vi "Thorlabs Translation Stage Module.vi"(7 "Action":T1, 8 "error in (no error)":errorcluster, 9 "Cluster In":T3, 10 "Set/Get":T2, 11 ".NET Refnum in":refnum<k24>) -> (0 "error out":errorcluster, 2 "Cluster out":T3, 3 ".NET Refnum out":refnum<k24>)   [LabVIEW 2018]
uses:
  C:/Project/SerialSectOCT/SerialSectOCT/Software/Thorlabs.MotionControl.Controls.dll
  Thorlabs.MotionControl.Controls.dll
  Hardware Mfg/Thorlabs Translation Stages/Controls/Translation Stage Cluster.ctl
  Controls/Translation Stage Types.ctl
  Controls/Set Get Controls.ctl
  Hardware Mfg/Thorlabs Translation Stages/Controls/Motion Translation Module Control.ctl
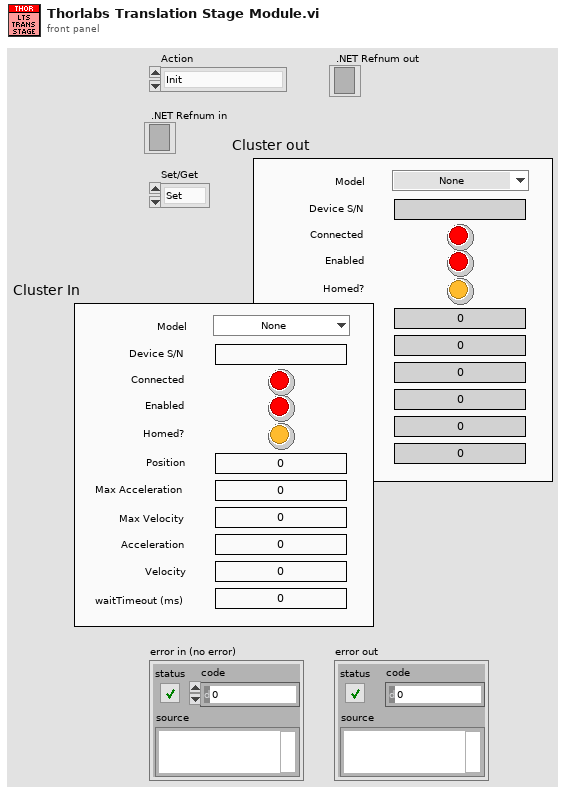
[diagram p1: front panel]
types:
  T1 = typedef "Motion Translation Module Control.ctl" = enum16{"Init", "Home", "Status", "Velocity/Accel", "Position", "Jog", "Stop", "Uninit", "Enable", "Disable"}
  T2 = typedef "Set Get Controls.ctl" = enum16{"Set", "Get"}
  T3 = typedef "Translation Stage Cluster.ctl" = cluster{"Position":dbl, "Is.Enabled?":bool, "Is.Connected?":bool, "Device SN":string, "AccelerationMaximum":dbl, "VelocityMaximum":dbl, "Acceleration":dbl, "Velocity":dbl, "waitTimeout (ms)":i32, "Model":T4, "Is.Homed?":bool}
  T4 = typedef "Translation Stage Types.ctl" = enum16{"None", "Thorlabs LTS", "Thorlabs MLJ"}
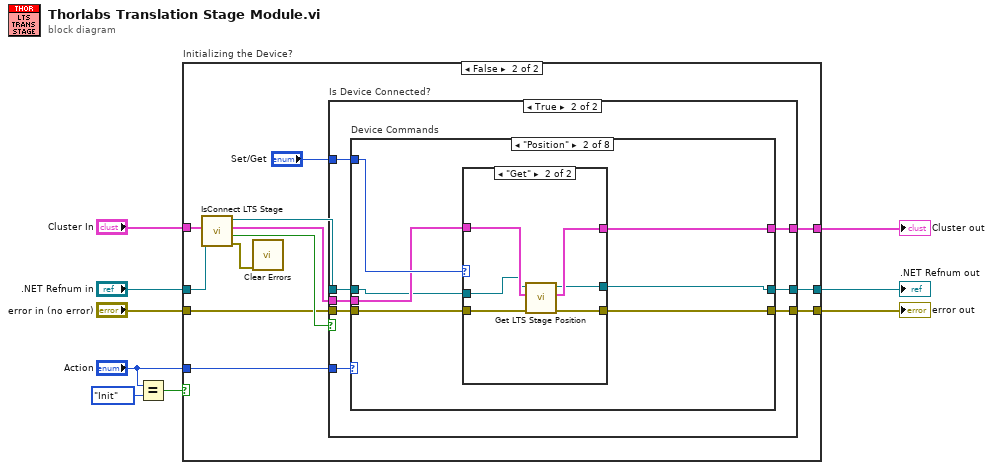
[diagram p0: block diagram]
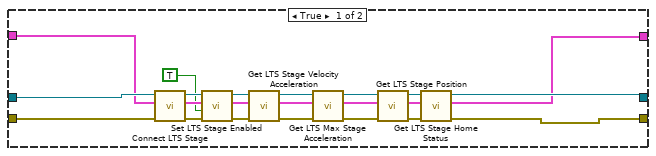
[diagram p2: hidden frame]
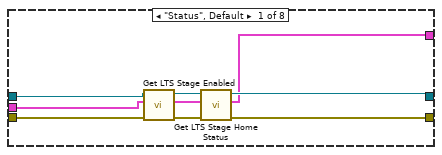
[diagram p4: hidden frame]
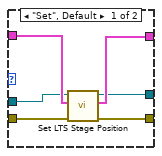
[diagram p5: hidden frame]
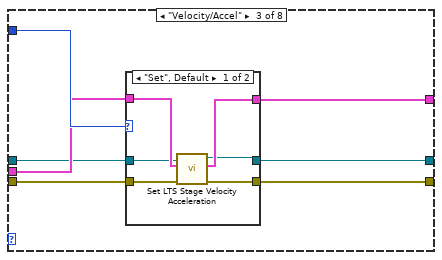
[diagram p6: hidden frame]
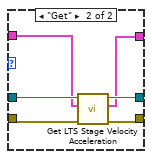
[diagram p7: hidden frame]
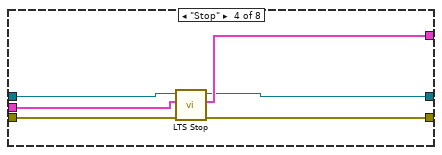
[diagram p8: hidden frame]
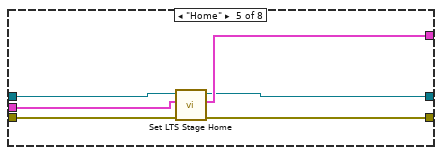
[diagram p9: hidden frame]
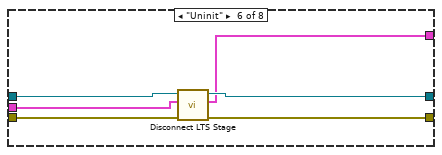
[diagram p10: hidden frame]
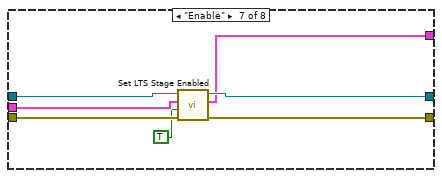
[diagram p11: hidden frame]
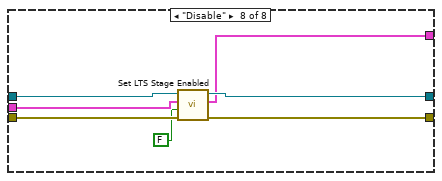
[diagram p12: hidden frame]
diagram:
  n1 = Equal?(x="Action", y=Motion_Translation_Module_Control."Init") -> (x = y?=w1:bool)
  n2 = case "Initializing the Device?" shown="False" w1 {
    tunnel: ".NET Refnum in" -> [w31 w38]
    tunnel: [w19 w43] -> w8
    tunnel: [w18 w42] -> w7
    tunnel: [w11 w41] -> w6
    tunnel: "error in (no error)" -> [w10 w33]
    tunnel: "Cluster In" -> [w30 w35]
    tunnel: "Action" -> [_ w40]
    frame True {
      n3 = call "Connect LTS Stage.vi"("error in (no error)"=w10, "Cluster in"=w30, "LTS Reference In"=w31) -> ("error out"=w29:errorcluster, "Cluster out"=w27:T3, "LTS Reference Out"=w28:refnum<k24>)  [unwired: 5 in, 1 out]
      n4 = call "Set LTS Stage Enabled.vi"("error in (no error)"=w29, "Enable?"=TRUE, "Cluster in"=w27, "LTS Reference In"=w28) -> ("error out"=w26:errorcluster, "Cluster out"=w25:T3, "LTS Reference Out"=w24:refnum<k24>)  [unwired: 5 in]
      n5 = call "Get LTS Stage Velocity Acceleration.vi"("error in (no error)"=w26, "Cluster in"=w25, "LTS Reference In"=w24) -> ("error out"=w23:errorcluster, "Cluster out"=w15:T3, "LTS Reference Out"=w14:refnum<k24>)  [unwired: 5 in, 1 out]
      n6 = call "Get LTS Max Stage Acceleration.vi"("error in (no error)"=w23, "Cluster in"=w15, "LTS Reference In"=w14) -> ("error out"=w16:errorcluster, "Cluster out"=w12:T3, "LTS Reference Out"=w13:refnum<k24>)  [unwired: 4 in, 2 out]
      n7 = call "Get LTS Stage Position.vi"("error in (no error)"=w16, "Cluster in"=w12, "LTS Reference In"=w13) -> ("error out"=w22:errorcluster, "Cluster out"=w21:T3, "LTS Reference Out"=w20:refnum<k24>)  [unwired: 5 in, 1 out]
      n8 = call "Get LTS Stage Home Status.vi"("error in (no error)"=w22, "Cluster in"=w21, "LTS Reference In"=w20) -> ("error out"=w11:errorcluster, "Cluster out"=w18:T3, "LTS Reference Out"=w19:refnum<k24>)  [unwired: 6 in]
    }
    frame False {
      n9 = call "IsConnect LTS Stage.vi"("Cluster in"=w35, "LTS Reference In"=w38) -> ("error out"=w32:errorcluster, "IsConnected"=w36:bool, "Cluster out"=w34:T3, "LTS Reference Out"=w37:refnum<k24>)  [unwired: 6 in]
      n10 = call <vilib>:"Clear Errors.vi"("error in (no error)"=w32) -> ()  [unwired: 5 in, 2 out]
      n11 = case "Is Device Connected?" shown="True" w36 {
        tunnel: w37 -> [w44 w54]
        tunnel: [w44 w53] -> w43
        tunnel: [w46 w52] -> w42
        tunnel: [w45 w51] -> w41
        tunnel: w33 -> [w45 w50]
        tunnel: "Set/Get" -> [_ w49]
        tunnel: w40 -> [_ w48]
        tunnel: w34 -> [w46 w47]
        frame False {
        }
        frame True {
          n12 = case "Device Commands" shown="\"Position\"" w48 {
            tunnel: w49 -> [_ w70 w89 _ _ _ _ _]
            tunnel: w47 -> [w56 w67 w86 w105 w111 w116 w123 w130]
            tunnel: w50 -> [w57 w69 w88 w107 w113 w119 w126 w133]
            tunnel: [w60 w65 w84 w103 w109 w117 w124 w131] -> w53
            tunnel: [w61 w68 w87 w106 w112 w118 w125 w132] -> w51
            tunnel: [w58 w66 w85 w104 w110 w115 w122 w129] -> w52
            tunnel: w54 -> [w55 w64 w83 w102 w108 w114 w121 w128]
            frame "Status", Default {
              n13 = call "Get LTS Stage Enabled.vi"("error in (no error)"=w57, "Cluster in"=w56, "LTS Reference In"=w55) -> ("error out"=w63:errorcluster, "Cluster out"=w59:T3, "LTS Reference Out"=w62:refnum<k24>)  [unwired: 5 in, 1 out]
              n14 = call "Get LTS Stage Home Status.vi"("error in (no error)"=w63, "Cluster in"=w59, "LTS Reference In"=w62) -> ("error out"=w61:errorcluster, "Cluster out"=w58:T3, "LTS Reference Out"=w60:refnum<k24>)  [unwired: 6 in]
            }
            frame "Position" {
              n15 = case shown="\"Get\"" w70 {
                tunnel: w69 -> [w76 w82]
                tunnel: [w75 w81] -> w68
                tunnel: w67 -> [w74 w80]
                tunnel: [w73 w79] -> w66
                tunnel: w64 -> [w72 w78]
                tunnel: [w71 w77] -> w65
                frame "Set", Default {
                  n16 = call "Set LTS Stage Position.vi"("error in (no error)"=w76, "Cluster in"=w74, "LTS Reference In"=w72) -> ("error out"=w75:errorcluster, "Cluster out"=w73:T3, "LTS Reference Out"=w71:refnum<k24>)  [unwired: 6 in]
                }
                frame "Get" {
                  n17 = call "Get LTS Stage Position.vi"("error in (no error)"=w82, "Cluster in"=w80, "LTS Reference In"=w78) -> ("error out"=w81:errorcluster, "Cluster out"=w79:T3, "LTS Reference Out"=w77:refnum<k24>)  [unwired: 5 in, 1 out]
                }
              }
            }
            frame "Velocity/Accel" {
              n18 = case shown="\"Set\", Default" w89 {
                tunnel: w88 -> [w95 w101]
                tunnel: [w94 w100] -> w87
                tunnel: w86 -> [w92 w97]
                tunnel: [w93 w96] -> w85
                tunnel: w83 -> [w91 w98]
                tunnel: [w90 w99] -> w84
                frame "Set", Default {
                  n19 = call "Set LTS Stage Velocity Acceleration.vi"("error in (no error)"=w95, "Cluster in"=w92, "LTS Reference In"=w91) -> ("error out"=w94:errorcluster, "Cluster out"=w93:T3, "LTS Reference Out"=w90:refnum<k24>)  [unwired: 6 in]
                }
                frame "Get" {
                  n20 = call "Get LTS Stage Velocity Acceleration.vi"("error in (no error)"=w101, "Cluster in"=w97, "LTS Reference In"=w98) -> ("error out"=w100:errorcluster, "Cluster out"=w96:T3, "LTS Reference Out"=w99:refnum<k24>)  [unwired: 5 in, 1 out]
                }
              }
            }
            frame "Stop" {
              n21 = call "LTS Stop.vi"("error in (no error)"=w107, "Cluster in"=w105, "LTS Reference In"=w102) -> ("error out"=w106:errorcluster, "Cluster out"=w104:T3, "LTS Reference Out"=w103:refnum<k24>)  [unwired: 6 in]
            }
            frame "Home" {
              n22 = call "Set LTS Stage Home.vi"("error in (no error)"=w113, "Cluster in"=w111, "LTS Reference In"=w108) -> ("error out"=w112:errorcluster, "Cluster out"=w110:T3, "LTS Reference Out"=w109:refnum<k24>)  [unwired: 6 in]
            }
            frame "Uninit" {
              n23 = call "Disconnect LTS Stage.vi"("error in (no error)"=w119, "Cluster in"=w116, "LTS Reference In"=w114) -> ("error out"=w118:errorcluster, "Cluster out"=w115:T3, "LTS Reference Out"=w117:refnum<k24>)  [unwired: 6 in]
            }
            frame "Enable" {
              n24 = call "Set LTS Stage Enabled.vi"("error in (no error)"=w126, "Enable?"=TRUE, "Cluster in"=w123, "LTS Reference In"=w121) -> ("error out"=w125:errorcluster, "Cluster out"=w122:T3, "LTS Reference Out"=w124:refnum<k24>)  [unwired: 5 in]
            }
            frame "Disable" {
              n25 = call "Set LTS Stage Enabled.vi"("error in (no error)"=w133, "Enable?"=FALSE, "Cluster in"=w130, "LTS Reference In"=w128) -> ("error out"=w132:errorcluster, "Cluster out"=w129:T3, "LTS Reference Out"=w131:refnum<k24>)  [unwired: 5 in]
            }
          }
        }
      }
    }
  }
  ".NET Refnum out" <- w8
  "Cluster out" <- w7
  "error out" <- w6
